vi "Select Data. (SUb VI)vi.vi"(8 "error in (no error)":errorcluster, 9 "input 1":string, 10 "Boolean":bool, 11 "Refnum in":T2) -> (0 "error out 2":errorcluster, 1 "recordset data":variant[][](array[variant]), 2 "resulting string":string, 3 "Refnum out":T2, 5 "recordset reference out":T1)   [LabVIEW 2024]
uses:
  <vilib>/addons/database/Connection.llb/Conn ObjectReference.ctl
  <vilib>/addons/database/Recordset.llb/Rec ObjectReference.ctl
  <vilib>/addons/database/Connection.llb/Conn Execute.vi
  <vilib>/addons/database/Recordset.llb/Rec Fetch Recordset Data (R).vi
  <vilib>/addons/database/NI_Database_API.lvlib
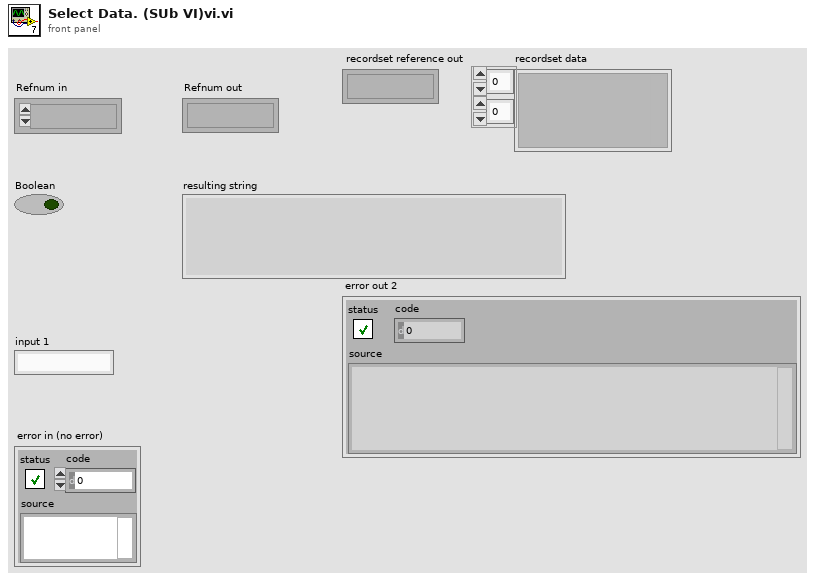
[diagram p1: front panel]
types:
  T1 = typedef "NI_Database_API.lvlib/Rec ObjectReference.ctl" = refnum<k1>
  T2 = typedef "NI_Database_API.lvlib/Conn ObjectReference.ctl" = refnum<k1>
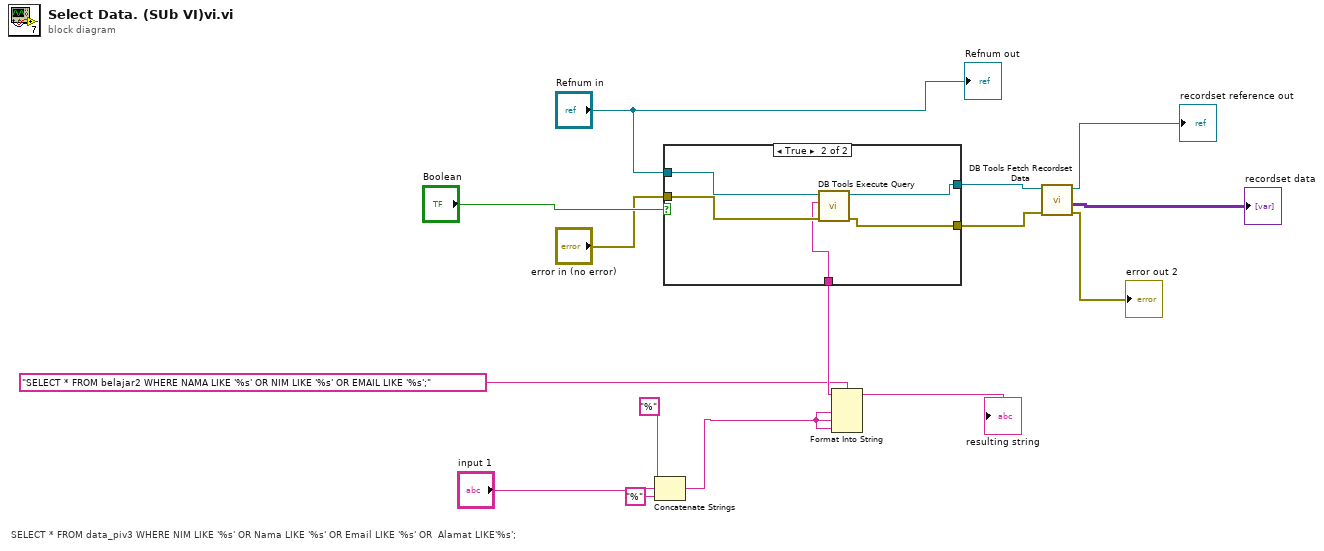
[diagram p0: block diagram]
diagram:
  # "SELECT * FROM data_piv3 WHERE NIM LIKE '%s' OR Nama LIKE '%s' OR Email LIKE '%s' OR  Alamat LIKE'%s';"
  n1 = Concatenate Strings("%" ("string"), "input 1", "%" ("string")) -> (w6:string)
  n2 = Format Into String(format string="SELECT * FROM belajar2 WHERE NAMA LIKE '%s' OR NIM LIKE '%s' OR EMAIL LIKE '%s';", w6, w6, w6) -> (resulting string=w12:string)  [unwired: 2 in, 1 out]
  "resulting string" <- w12
  n3 = case shown="True" "Boolean" {
    tunnel: "Refnum in" -> [_ w20]
    tunnel: "error in (no error)" -> [w15 w19]
    tunnel: w12 -> [_ w18]
    tunnel: [w15 w17] -> w5
    tunnel: [_ w16] -> w4
    frame False {
    }
    frame True {
      n4 = call-poly <vilib>:"DB Tools Execute Query.vi"("error in (no error)"=w19, "SQL query"=w18, "connection reference"=w20) -> ("error out"=w17:errorcluster, "recordset reference"=w16:T1)  [unwired: 5 in]
    }
  }
  n5 = call-poly <vilib>:"DB Tools Fetch Recordset Data.vi"("error in (no error)"=w5, "recordset reference"=w4) -> ("error out"=→"error out 2":errorcluster, "recordset data"=→"recordset data":variant[][], "recordset reference out"=→"recordset reference out":T1)  [unwired: 3 in]
  "Refnum out" <- "Refnum in"
